vi "Determine Message Type.vi"(8 "error in":errorcluster, 10 "data in":string) -> (0 "error out":errorcluster, 2 "message type":T1, 3 "stripped message":string)   [LabVIEW 2013, in "NATS Core.lvlib"]
doc: "Determines the type of message received from the NATS server. Strips off message pre/postamble for type-identified messages when appropriate."
uses:
  NATS Core.lvlib
  Controls/msg type.ctl
  <vilib>/Utility/error.llb/whitespace.ctl
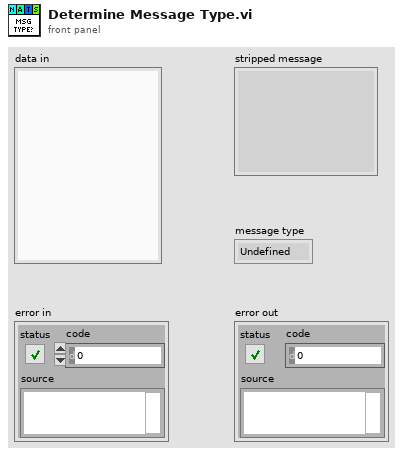
[diagram p1: front panel]
types:
  T1 = typedef "NATS Core.lvlib/msg type.ctl" = enum16{"Undefined", "MSG", "HMSG", "+OK", "PING", "PONG", "-ERR", "INFO"}
  T2 = typedef "whitespace.ctl" = u16
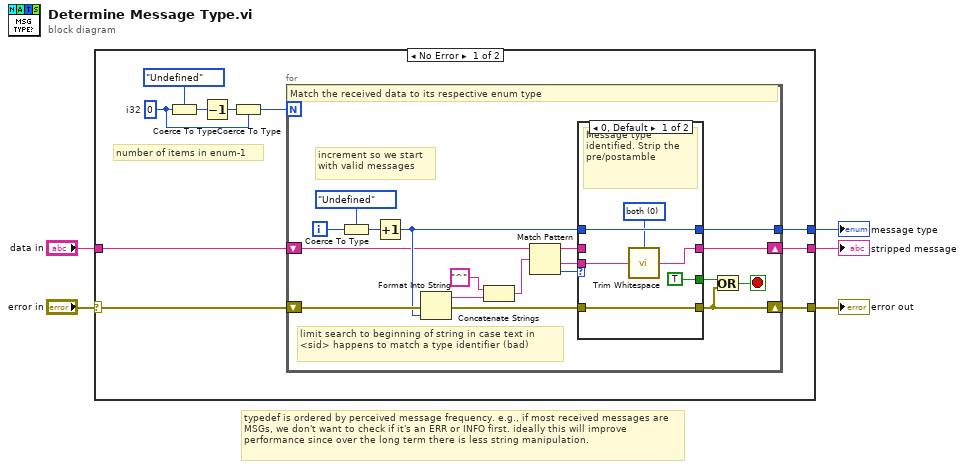
[diagram p0: block diagram]
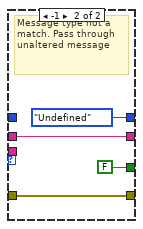
[diagram p2: hidden frame]
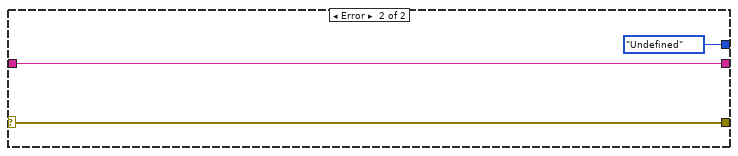
[diagram p3: hidden frame]
diagram:
  # "typedef is ordered by perceived message frequency. e.g., if most received messages are MSGs, we don't want to check if it's an ERR or INFO first. ideally this will improve performance since over the long term there is less string manipulation."
  n1 = case shown="No Error" "error in" {
    selector: "error in" -> [w13 w44]
    tunnel: "data in" -> [w15 w46]
    tunnel: [w14 w44] -> w4
    tunnel: [w7 msg_type."Undefined" ("message type")] -> w2
    tunnel: [w6 w46] -> w1
    frame No Error {
      w9 = 0  # i32
      # "number of items in enum-1"
      n2 = Coerce To Type(0:w9, 1:msg_type."Undefined" ("message type")) -> (2:w11:T1)
      n3 = Decrement(x=w11) -> (x-1=w10:T1)
      n4 = Coerce To Type(0:w10, 1:w9) -> (2:w8:i32)
      n5 = for {
        N: w8 -> [_]
        shift-right: [w30] -> w14
        shift-left: w13 -> [w28]
        tunnel: [w33] -> w7
        shift-right: [w22] -> w6
        shift-left: w15 -> [w21]
        i -> [w25]
        stop <- w29 stop-if-true
        # "limit search to beginning of string in case text in <sid> happens to match a type identifier (bad)"
        # "increment so we start with valid messages"
        # "Match the received data to its respective enum type"
        n6 = Coerce To Type(0:w25, 1:msg_type."Undefined" ("message type")) -> (2:w24:T1)
        n7 = Increment(x=w24) -> (x+1=w23:T1)
        n8 = Format Into String(error in=w28, w23) -> (resulting string=w18:string, error out=w27:errorcluster)  [unwired: 2 in]
        n9 = Concatenate Strings("^" ("string"), w18) -> (w16:string)
        n10 = Match Pattern(string=w21, regular expression=w16) -> (before substring=w20:string, after substring=w19:string, offset past match=w32:i32)  [unwired: 1 in, 1 out]
        n11 = case shown="0, Default" w32 {
          tunnel: w27 -> [w37 w43]
          tunnel: [w37 w43] -> w30
          tunnel: [w38 msg_type."Undefined" ("message type")] -> w33
          tunnel: w23 -> [w38 _]
          tunnel: [TRUE FALSE] -> w31
          tunnel: w19 -> [w36 _]
          tunnel: [w35 w40] -> w22
          tunnel: w20 -> [_ w40]
          frame 0, Default {
            w34 = T2 0 items=["both", "start of string", "end of string"] ("location (both)")
            # "Message type identified. Strip the pre/postamble"
            n12 = call <vilib>:"Trim Whitespace.vi"("string"=w36, "location (both)"=w34) -> ("trimmed string"=w35:string)
          }
          frame -1 {
            # "Message type not a match. Pass through unaltered message"
          }
        }
        n13 = Or(x=w31, y=w30) -> (x .or. y?=w29:bool)
      }
    }
    frame Error {
    }
  }
  "error out" <- w4
  "message type" <- w2
  "stripped message" <- w1
